vi "Load MPLOT.vi"(8 "error in (no error)":errorcluster, 11 "Filepath":path) -> (0 "error out":errorcluster, 3 "RocketPlots":T1[](array[typedef]) {"RocketPlotConfig"."General"."Time to Plot" format="%<%M:%S>t"; "Plot Bounds (%)"."Bottom (%)" format="%.2f"; "Plot Bounds (%)"."Top (%)" format="%.2f"; "Plot Bounds (%)"."Right (%)" format="%.2f"; "Plot Bounds (%)"."Left (%)" format="%.2f"})   [LabVIEW 2021, in "MultiStokePlot.lvlib" / "MultiPlotPanel.lvclass"]
uses:
  MultiPlotPanel/MultiPlotPanel.lvclass
  SinglePlotConfig.ctl
  SubVIs/Window Position.ctl
  <userlib>/bjustice/RocketPlot/TypeDefs/plot load data V2.ctl
  <userlib>/bjustice/RocketPlot/TypeDefs/plot properties V2.ctl
  <userlib>/bjustice/RocketPlot/TypeDefs/plot attributes V2.ctl
  <userlib>/bjustice/RocketPlot/TypeDefs/Plot scale axis properties.ctl
  <userlib>/bjustice/RocketPlot/TypeDefs/Plot general properties.ctl
  230cbe50-02c9-41a1-a09f-b1b8e06de6a4.vi
  <vilib>/JDP Science/JSONtext/JSON text to Variant.vi
  <vilib>/JDP Science/JSONtext/LVClass Serializer/JSONtext LVClass Serializer.lvclass
  <userlib>/bjustice/RocketPlot/RocketPlot.lvlib
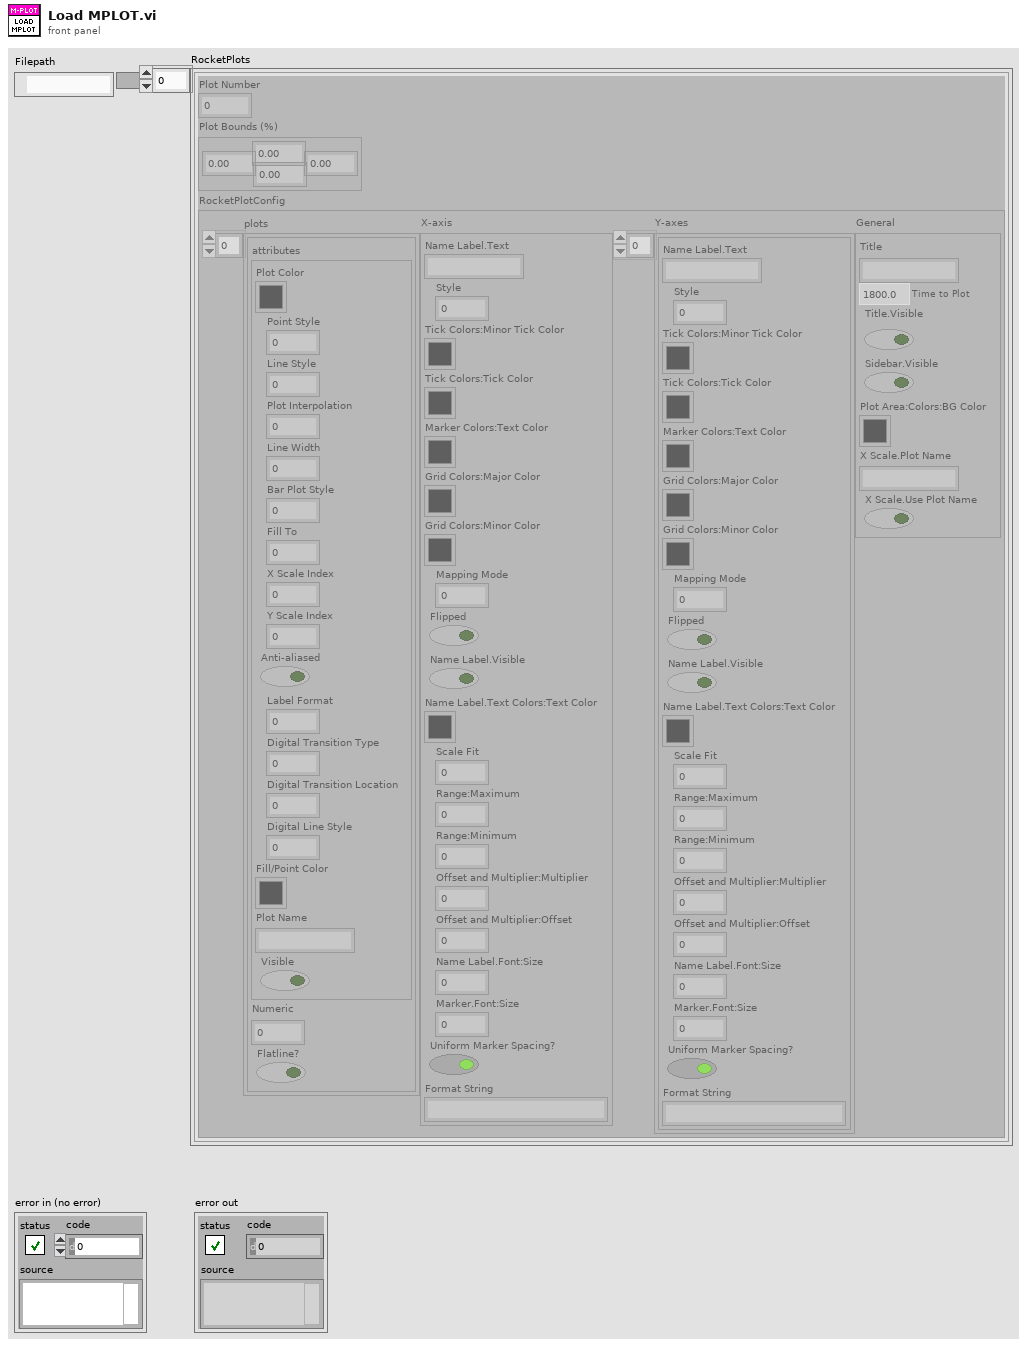
[diagram p1: front panel]
types:
  T1 = typedef "MultiStokePlot.lvlib/MultiPlotPanel.lvclass/SinglePlotConfig.ctl" = cluster{"Plot Number":i32, "Plot Bounds (%)":T2, "RocketPlotConfig":T3}
  T2 = typedef "MultiStokePlot.lvlib/MultiPlotPanel.lvclass/Window Position.ctl" = cluster{"Left (%)":dbl, "Top (%)":dbl, "Right (%)":dbl, "Bottom (%)":dbl}
  T3 = typedef "RocketPlot.lvlib/plot load data V2.ctl" = cluster{"plots":T4[], "X-axis":T6, "Y-axes":T6[], "General":T7}
  T4 = typedef "RocketPlot.lvlib/plot properties V2.ctl" = cluster{"attributes":T5, "Numeric":dbl, "Flatline?":bool}
  T5 = typedef "RocketPlot.lvlib/plot attributes V2.ctl" = cluster{"Plot Color":u32, "Point Style":u8, "Line Style":u8, "Plot Interpolation":u8, "Line Width":u8, "Bar Plot Style":u8, "Fill To":i16, "X Scale Index":u32, "Y Scale Index":u32, "Anti-aliased":bool, "Label Format":u8, "Digital Transition Type":u8, "Digital Transition Location":u8, "Digital Line Style":u8, "Fill/Point Color":u32, "Plot Name":string, "Visible":bool}
  T6 = typedef "RocketPlot.lvlib/Plot scale axis properties.ctl" = cluster{"Name Label.Text":string, "Style":u8, "Tick Colors:Minor Tick Color":u32, "Tick Colors:Tick Color":u32, "Marker Colors:Text Color":u32, "Grid Colors:Major Color":u32, "Grid Colors:Minor Color":u32, "Mapping Mode":u8, "Flipped":bool, "Name Label.Visible":bool, "Name Label.Text Colors:Text Color":u32, "Scale Fit":u8, "Range:Maximum":dbl, "Range:Minimum":dbl, "Offset and Multiplier:Multiplier":dbl, "Offset and Multiplier:Offset":dbl, "Name Label.Font:Size":u32, "Marker.Font:Size":u32, "Uniform Marker Spacing?":bool, "Format String":string}
  T7 = typedef "RocketPlot.lvlib/Plot general properties.ctl" = cluster{"Title":string, "Time to Plot":dbl, "Title.Visible":bool, "Sidebar.Visible":bool, "Plot Area:Colors:BG Color":u32, "X Scale.Plot Name":string, "X Scale.Use Plot Name":bool}
  T8 = enum16{"open", "replace", "create", "open or create", "replace or create", "replace or create with confirmation"}
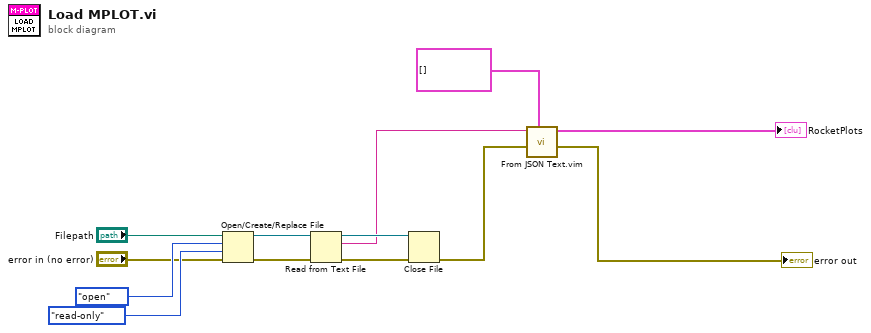
[diagram p0: block diagram]
diagram:
  n1 = Open/Create/Replace File(file path (use dialog)="Filepath", error in="error in (no error)", operation (0:open)=T8."open", access (0:read/write)=enum16{"read/write", "read-only", "write-only"}."read-only") -> (refnum out=w12:refnum<file>, error out=w10:errorcluster)  [unwired: 2 in, 1 out]
  n2 = Read from Text File(file (use dialog)=w12, error in=w10) -> (refnum out=w11:refnum<file>, text=w2:string, error out=w9:errorcluster)  [unwired: 2 in, 1 out]
  n3 = Close File(refnum=w11, error in=w9) -> (error out=w5:errorcluster)  [unwired: 1 out]
  n4 = call "From JSON Text.vim"("Data Type and Default Value"=T1[] [] ("Array"), "error in (no error)"=w5, "JSON"=w2) -> ("error out"=→"error out":errorcluster, "Data out"=→"RocketPlots":T1[])  [unwired: 7 in]
